vi "Process Beam data.vi"(8 "error in (no error)":errorcluster, 10 "Expose to beam":bool, 11 "Beam in":refnum<class "Beam.lvclass">) -> (0 "error out":errorcluster, 3 "Beam out":refnum<class "Beam.lvclass">)   [LabVIEW 2019, in "Beam.lvclass"]
uses:
  Beam.lvclass
  Beam.lvclass/Beam.ctl
panel:
  in  "BOS":dbl
  in  "EOS":dbl
  in  "Spill ID":dbl
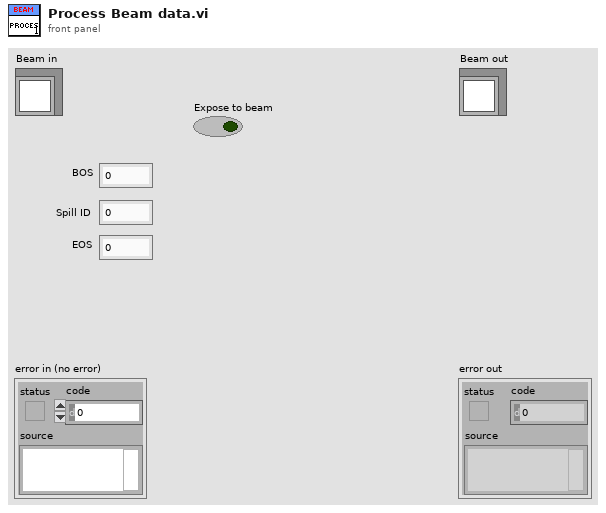
[diagram p1: front panel]
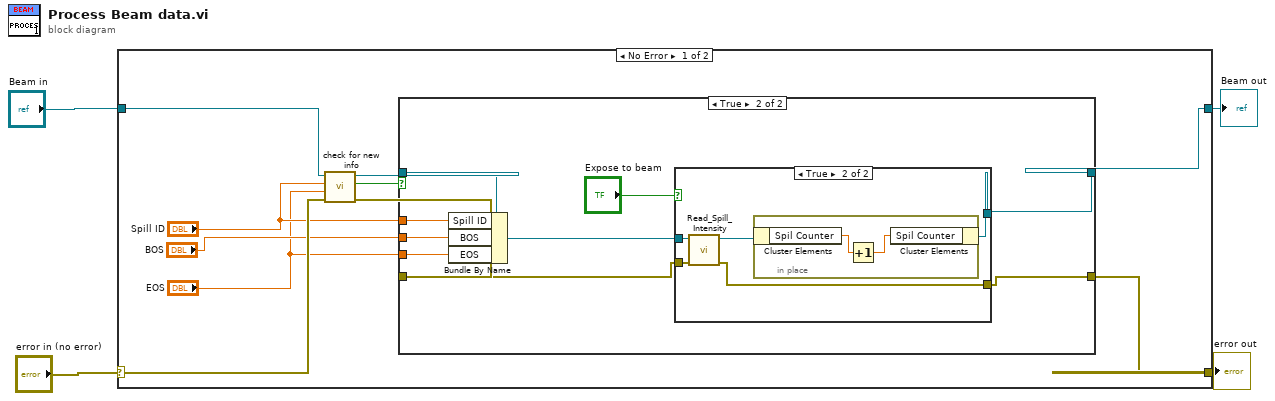
[diagram p0: block diagram]
diagram:
  n1 = case shown="No Error" "error in (no error)" {
    selector: "error in (no error)" -> [w13 w36]
    tunnel: [w6 w36] -> w3
    tunnel: [w5 w35] -> w1
    tunnel: "Beam in" -> [w14 w35]
    frame No Error {
      n2 = call "check for new info.vi"("error in (no error)"=w13, "EOS"="EOS", "Spill ID"="Spill ID", "Beam in"=w14) -> ("error out"=w7:errorcluster, "New Spill recieved"=w12:bool, "Beam out"=w11:refnum<class "Beam.lvclass">)  [unwired: 4 in, 1 out]
      n3 = case shown="True" w12 {
        tunnel: w11 -> [w16 w25]
        tunnel: "Spill ID" -> [_ w24]
        tunnel: "BOS" -> [_ w23]
        tunnel: "EOS" -> [_ w22]
        tunnel: w7 -> [w15 w21]
        tunnel: [w16 w19] -> w5
        tunnel: [w15 w18] -> w6
        frame False {
        }
        frame True {
          n4 = Bundle By Name(cluster=w25, "Spill ID"=w24, "BOS"=w23, "EOS"=w22) -> (w20:refnum<class "Beam.lvclass">)
          n5 = case shown="True" "Expose to beam" {
            tunnel: w21 -> [w26 w32]
            tunnel: w20 -> [w27 w31]
            tunnel: [w27 w29] -> w19
            tunnel: [w26 w28] -> w18
            frame False {
            }
            frame True {
              n6 = call "Read_Spill_Intensity.vi"("error in (no error)"=w32, "Beam in"=w31) -> ("error out"=w28:errorcluster, "Beam out"=w30:refnum<class "Beam.lvclass">)  [unwired: 8 in]
              n7 = in-place {
                n8 = in-place-cluster #1(w30) -> ("Spil Counter"=w34:dbl)
                n9 = Increment(x=w34) -> (x+1=w33:dbl)
                n10 = in-place-cluster #1("Spil Counter"=w33) -> (w29:refnum<class "Beam.lvclass">)
              }
            }
          }
        }
      }
    }
    frame Error {
    }
  }
  "error out" <- w3
  "Beam out" <- w1
